vi "opencvSegmentConvertCoordinates.vi"   [LabVIEW 2017]
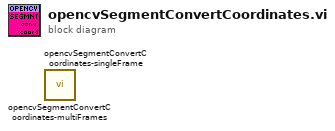
[diagram p0: block diagram]
diagram:
  n1 = call "opencvSegmentConvertCoordinates-multiFrames.vi"() -> ()  [unwired: 3 in, 1 out]
  n2 = call "opencvSegmentConvertCoordinates-singleFrame.vi"() -> ()  [unwired: 3 in, 1 out]
